vi "Set_4275_Configuration.vi"(8 "error in":errorcluster, 11 "Keystate":string) -> (0 "error out":errorcluster)   [LabVIEW 2020]
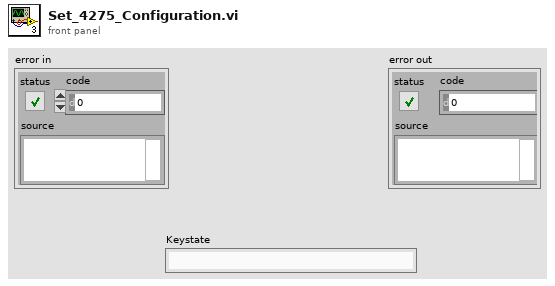
[diagram p1: front panel]
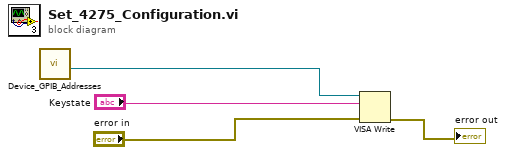
[diagram p0: block diagram]
diagram:
  n1 = call "Device_GPIB_Addresses.vi"() -> ("HP 4275A Address"=w1:refnum<visa-resource-name>)  [unwired: 9 in, 2 out]
  n2 = VISA Write(VISA resource name=w1, write buffer="Keystate", error in (no error)="error in") -> (error out=→"error out":errorcluster)  [unwired: 2 out]
